vi "AlliGator Display True Phasor Plot Value.vi"(7 "AlliGator Ctrl Refnums":T1, 8 "error in (no error)":errorcluster) -> (0 "error out":errorcluster)   [LabVIEW 2021, in "AlliGator Phasor Plot.lvlib"]
uses:
  AlliGator Phasor Plot.lvlib
  GUI/AlliGator Ctrl Refnums.ctl
  GUI/AlliGator Other Ctrl Refnums.ctl
  GUI/AlliGator State Indicator.ctl
  GUI/AlliGator Main Window Tabs.ctl
  GUI/AlliGator Phasor Plot Ctrl Refnums.ctl
  GUI/AlliGator Phasor Graph Ctrl Refnums.ctl
  Phasor/Phasor Calibration Type.ctl
  GUI/AlliGator Dataset Ctrl Refnums.ctl
  Source Image/AlliGator Displayed Image.ctl
  GUI/AlliGator Registered Events Ctrl Refnums.ctl
  GUI/AlliGator Image Histogram Control Refnums.ctl
  Histograms/Linear Histogram Options.ctl
  Histograms/Histogram Bin Option.ctl
  Histograms/Histogram Bin Position.ctl
  Decay Fit Parameter Map/AlliGator Decay Fit Map Control Refnums.ctl
  Fits/IRF(X)PSED/Decay Fit Parameters & Derived Quantities List v2.ctl
  Parameter Map/AlliGator Parameter Map Control Refnums.ctl
  Source Image/AlliGator Source Image.lvlib
  Fits/Fits.lvlib
  GUI/AlliGator GUI.lvlib
  Phasor/Phasor.lvlib
  Histograms/Histogram Window.lvlib
  Decay Fit Parameter Map/AlliGator Decay Fit Parameter Map.lvlib
  Parameter Map/AlliGator Parameter Map.lvlib
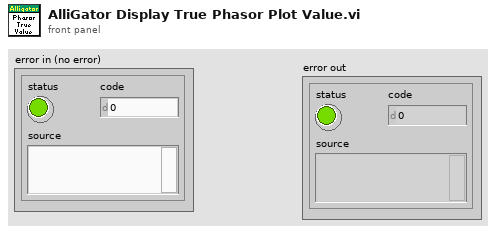
[diagram p1: front panel]
types:
  T1 = typedef "AlliGator GUI.lvlib/AlliGator Ctrl Refnums.ctl" = cluster{"Other AlliGator Ctrl Refnums":T2, "Phasor Plot Ctrl Refnums":T3, "Phasor Graph Ctrl Refnums":T4, "Dataset Control Refnums":T5, "Registered Events Ctrl Refnums":T6, "Image Histogram Ctrl Refnums":T7, "Decay Fit Map Ctrl Refnums":T8, "Parameter Map Ctrl Refnums":T9}
  T2 = typedef "AlliGator GUI.lvlib/AlliGator Other Ctrl Refnums.ctl" = cluster{"State Indicators":refnum<vi>, " Progress Bar":refnum<vi>, "Decay Graph Active":refnum<vi>, "Decay Statistics Bin":refnum<vi>, "Time Step":refnum<vi>, "Use File Timestamp":refnum<vi>, "Tab Control":refnum<vi>, "CPU":refnum<vi>, "Abort Fit":refnum<vi>, "Dataset File/Folder Path":refnum<vi>, "Abort ROI Creation":refnum<vi>, "Event LED":refnum<vi>, "Dataset File/Folder Path 2":refnum<vi>, "Dataset File/Folder Path 3":refnum<vi>, "Dataset File/Folder Path 4":refnum<vi>, "Dataset File/Folder Path 5":refnum<vi>, "Dataset File/Folder Path 6":refnum<vi>, "Dataset File/Folder Path 7":refnum<vi>, "Dataset File/Folder Path 8":refnum<vi>, "Dataset File/Folder Path 9":refnum<vi>, "Dataset File/Folder Path 10":refnum<vi>, "Dataset File/Folder Path 11":refnum<vi>}
  T3 = typedef "AlliGator GUI.lvlib/AlliGator Phasor Plot Ctrl Refnums.ctl" = cluster{"Phasor Ratio":refnum<vi>, "Modulus Lifetime":refnum<vi>, "Phasor at cursor (m, phi)":refnum<vi>, "Phase Lifetime":refnum<vi>, "Phasor at cursor (g, s)":refnum<vi>, "Phasor Plor Average Lifetime":refnum<vi>, "Phasor Plot Active":refnum<vi>, "Save Phasor Plot":refnum<vi>, "Image Overlay Color":refnum<vi>, "Phasor Plot Color Scale":refnum<vi>, "Reference 1 Button":refnum<vi>, "Reference 2 Button":refnum<vi>, "True Phasor Plot Value":refnum<vi>}
  T4 = typedef "AlliGator GUI.lvlib/AlliGator Phasor Graph Ctrl Refnums.ctl" = cluster{"Phasor Ratio":refnum<vi>, "Modulus Lifetime":refnum<vi>, "Phasor at cursor (m, phi)":refnum<vi>, "Phase Lifetime":refnum<vi>, "Phasor at cursor (g, s)":refnum<vi>, "Phasor Graph Average Lifetime":refnum<vi>, "Phasor Graph Active":refnum<vi>, "Save Phasor Graph":refnum<vi>, "Phasor Frame Slide":refnum<vi>, "Single Step Phasor":refnum<vi>, "Calibration Type":refnum<vi>, "Show Line":refnum<vi>, "Phase Lifetime 1":refnum<vi>, "Phase Lifetime 2":refnum<vi>, "Phasor Graph Frequency":refnum<vi>, "Phasor Reference 1 Control":refnum<vi>, "Phasor Reference 2 Control":refnum<vi>, "Calibration Lifetime":refnum<vi>, "Phase Lifetime SDV":refnum<vi>, "Average Lifetime SDV":refnum<vi>, "Phasor Ratio SDV":refnum<vi>, "Modulus Lifetime SDV":refnum<vi>}
  T5 = typedef "AlliGator GUI.lvlib/AlliGator Dataset Ctrl Refnums.ctl" = cluster{"Current Data":refnum<vi>, "Gate Image Slide":refnum<vi>, "Time Point Slide":refnum<vi>, "Current Time Stamp":refnum<vi>, "Save Image":refnum<vi>, "Displayed Image":refnum<vi>, "Overlay Mode":refnum<vi>, "Phasor Overlay Color":refnum<vi>, "Image Color Scale":refnum<vi>, "Use ROI as Search Area":refnum<vi>, "Source Image ROI Color":refnum<vi>, "True Pixel Value":refnum<vi>}
  T6 = typedef "AlliGator GUI.lvlib/AlliGator Registered Events Ctrl Refnums.ctl" = cluster{"Time Point Slider":refnum<vi>, "Phasor Plot Display Range":refnum<vi>, "Decay Graph":refnum<vi>, "Decay Statistics Graph":refnum<vi>, "Intensity Time Trace":refnum<vi>, "Phasor Graph":refnum<vi>, "Phasor Ratio Graph":refnum<vi>, "Lifetime Graph":refnum<vi>, "Phasor Plot Display":refnum<vi>, "Source Image Display":refnum<vi>, "Decay Fit Parameter Map Display Range":refnum<vi>, "Decay Fit Parameter Map Display":refnum<vi>, "Parameter Map Display Range":refnum<vi>, "Parameter Map Display":refnum<vi>, "Phasor Plot Display Range":refnum<vi>}
  T7 = typedef "AlliGator GUI.lvlib/AlliGator Image Histogram Control Refnums.ctl" = cluster{"Image Histogram":refnum<vi>, "Image Histogram Options":refnum<vi>, "Image Histogram Active":refnum<vi>, "Image Histogram Upper Percentile":refnum<vi>, "Image Histogram Lower Percentile":refnum<vi>, "Auto-Adjust Contrast":refnum<vi>}
  T8 = typedef "AlliGator Decay Fit Parameter Map.lvlib/AlliGator Decay Fit Map Control Refnums.ctl" = cluster{"Decay Fit Parameter Map Color Scale":refnum<vi>, "Decay Fit Parameter":refnum<vi>, "Max Parameter":refnum<vi>, "Min Parameter":refnum<vi>, "Decay Fit Parameter Map Display":refnum<vi>, "Decay Fit Parameter Map Display Range":refnum<vi>, "Decay Parameter Map X":refnum<vi>, "Decay Parameter Map Y":refnum<vi>, "Decay Parameter Map Value":refnum<vi>}
  T9 = typedef "AlliGator Parameter Map.lvlib/AlliGator Parameter Map Control Refnums.ctl" = cluster{"Parameter Map Color Scale":refnum<vi>, "Map Parameter":refnum<vi>, "Max Parameter":refnum<vi>, "Min Parameter":refnum<vi>, "Parameter Map Display":refnum<vi>, "Parameter Map Display Range":refnum<vi>, "Parameter Map Set":refnum<vi>, "Parameter Map X":refnum<vi>, "Parameter Map Y":refnum<vi>, "Parameter Map Value":refnum<vi>}
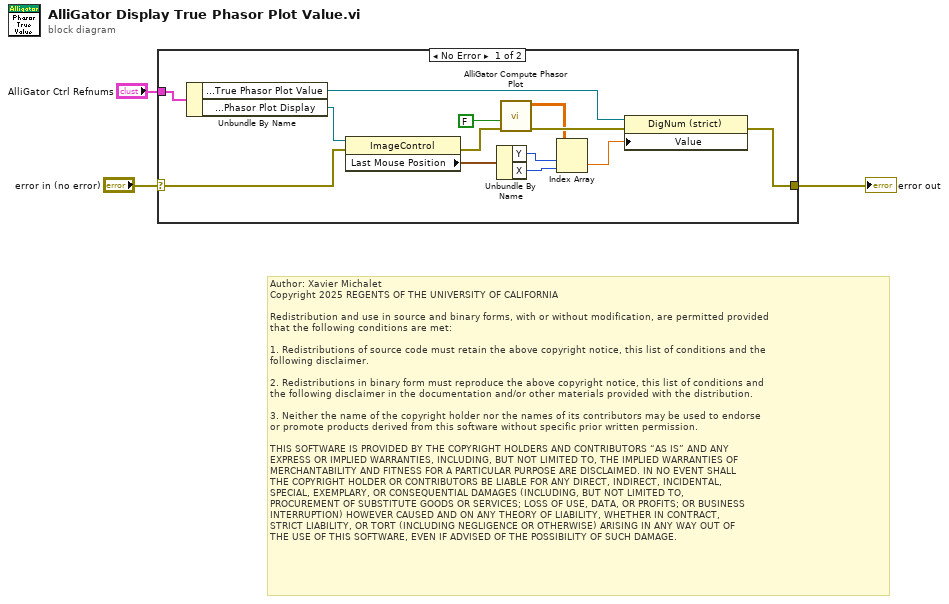
[diagram p0: block diagram]
diagram:
  # "Author: Xavier Michalet\nCopyright 2025 REGENTS OF THE UNIVERSITY OF CALIFORNIA\n\nRedistribution and use in source and binary forms, with or without modification, are permitted provided\nthat the following conditions are met:\n\n1. Redistributions of source code must retain the above copyright notice, this list of conditions and the\nfollowing disclaimer.\n\n2. Redistributions in binary form must reproduce the above copyright notice, this list of conditions and\nthe following disclaimer in the documentation and/or other materials provided with the distribution.\n\n3. Neither the name of the copyright holder nor the names of its contributors may be used to endorse \nor promote products derived from this software without specific prior written permission.\n\nTHIS SOFTWARE IS PROVIDED BY THE COPYRIGHT HOLDERS AND CONTRIBUTORS “AS IS” AND ANY \nEXPRESS OR IMPLIED WARRANTIES, INCLUDING, BUT NOT LIMITED TO, THE IMPLIED WARRANTIES OF\nMERCHANTABILITY AND FITNESS FOR A PARTICULAR PURPOSE ARE DISCLAIMED. IN NO EVENT SHALL\nTHE COPYRIGHT HOLDER OR CONTRIBUTORS BE LIABLE FOR ANY DIRECT, INDIRECT, INCIDENTAL, \nSPECIAL, EXEMPLARY, OR CONSEQUENTIAL DAMAGES (INCLUDING, BUT NOT LIMITED TO, \nPROCUREMENT OF SUBSTITUTE GOODS OR SERVICES; LOSS OF USE, DATA, OR PROFITS; OR BUSINESS\nINTERRUPTION) HOWEVER CAUSED AND ON ANY THEORY OF LIABILITY, WHETHER IN CONTRACT, \nSTRICT LIABILITY, OR TORT (INCLUDING NEGLIGENCE OR OTHERWISE) ARISING IN ANY WAY OUT OF\nTHE USE OF THIS SOFTWARE, EVEN IF ADVISED OF THE POSSIBILITY OF SUCH DAMAGE."
  n1 = case shown="No Error" "error in (no error)" {
    selector: "error in (no error)" -> [w6 w17]
    tunnel: "AlliGator Ctrl Refnums" -> [w16 _]
    tunnel: [w15 w17] -> w2
    frame No Error {
      n2 = Unbundle By Name(w16) -> ("Phasor Plot Ctrl Refnums.True Phasor Plot Value"=w14:refnum<vi>, "Registered Events Ctrl Refnums.Phasor Plot Display"=w8:refnum<vi>)
      n3 = property class="ImageControl"(reference=w8, error in=w6) -> (error out=w5:errorcluster, "Last Mouse Position"=w7:cluster{"X":i32, "Y":i32})  [unwired: 1 out]
      n4 = Unbundle By Name(w7) -> ("Y"=w13:i32, "X"=w9:i32)
      n5 = call "AlliGator Compute Phasor Plot.vi"("error in (no error)"=w5, "Compute Phasor Plot (F)"=FALSE ("Compute Phasor Plot")) -> ("error out"=w11:errorcluster, "Phasor Plot"=w10:sgl[][])  [unwired: 6 in, 2 out]
      n6 = Index Array(array=w10, index (row)=w13, index (col)=w9) -> (element=w12:sgl)
      n7 = property class="DigNum (strict)"(reference=w14, error in=w11, "Value"=w12) -> (error out=w15:errorcluster)  [unwired: 1 out]
    }
    frame Error {
    }
  }
  "error out" <- w2
